vi "ConfigureLevel.vi"(8 "error in (no error)":errorcluster, 11 "SpecAnBase in":refnum<class "SpecAnBase.lvclass">) -> (0 "error out":errorcluster, 3 "SpecAnBase out":refnum<class "SpecAnBase.lvclass">)   [LabVIEW 2014, in "SpecAnPlugins.lvlib" / "SpecAnBase.lvclass"]
doc: "This function configures the vertical attributes of the spectrum analyzer. This corresponds to the Amplitude Units, Input Attenuation, Input Impedance, Reference Level, and Reference Level Offset attributes."
uses:
  SpecAnBase.lvclass
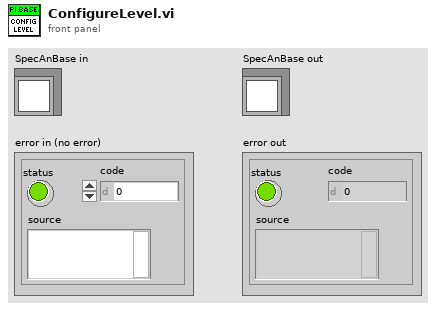
[diagram p1: front panel]
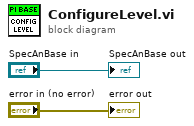
[diagram p0: block diagram]
diagram:
  "error out" <- "error in (no error)"
  "SpecAnBase out" <- "SpecAnBase in"
